vi "libssh2_channel_receive_window_adjust2.vi"(8 "error in (no error)":errorcluster, 9 "force (F)":bool, 10 "adjustment":u32, 11 "channel":T1) -> (0 "error out":errorcluster, 2 "window":u32)   [LabVIEW 2013, in "libssh2.lvlib"]
doc: "Adjust the receive window for a channel by <B>adjustment</B> bytes.\nIf the amount to be adjusted is less than 1024 and <B>force</B> is zero the adjustment amount will be queued for a later packet.\n\nReturns the new size of the receive window."
uses:
  libssh2.lvlib
  Channel Refnum.ctl
  Not A Channel.vi
  <vilib>/Utility/error.llb/Error Cluster From Error Code.vi
  Global Settings.vi
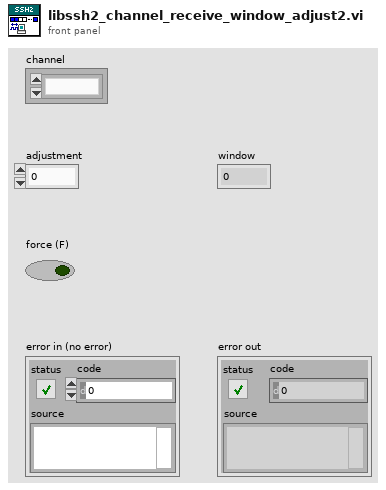
[diagram p1: front panel]
types:
  T1 = typedef "libssh2.lvlib/Channel Refnum.ctl" = refnum<k1>
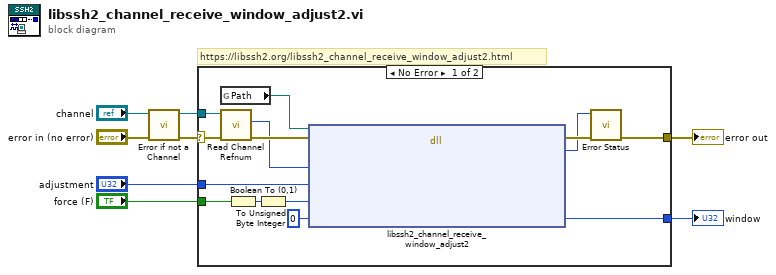
[diagram p0: block diagram]
diagram:
  # "https://libssh2.org/libssh2_channel_receive_window_adjust2.html"
  n1 = call "Error if not a Channel.vi"("error in (no error)"="error in (no error)", "channel"="channel") -> ("error out"=w6:errorcluster, "channel out"=w4:T1)  [unwired: 8 in]
  n2 = case shown="No Error" w6 {
    selector: w6 -> [w22 w23]
    tunnel: [w21 w23] -> w8
    tunnel: w4 -> [w20 _]
    tunnel: "adjustment" -> [w14 _]
    tunnel: "force (F)" -> [w13 _]
    tunnel: [w10 _] -> w1
    frame No Error {
      n3 = global read "Global Settings.vi" "Path"() -> (w16:path)
      n4 = call "Read Channel Refnum.vi"("error in (no error)"=w22, "channel"=w20) -> ("error out"=w18:errorcluster, "LIBSSH2_CHANNEL*"=w17:u64)  [unwired: 8 in]
      n5 = Boolean To (0,1)(Boolean=w13) -> (0, 1=w12:i16)
      n6 = To Unsigned Byte Integer(number=w12) -> (unsigned 8bit integer=w11:u8)
      n7 = dll-call lib="?" fn="libssh2_channel_receive_window_adjust2"(path in=w16, error in=w18, "channel"=w17, "adjustment"=w14, "force"=w11, "window"=u32 0) -> (error out=w19:errorcluster, "return value"=w15:i32, "window"=w10:u32)  [unwired: 4 in, 1 out]
      n8 = call "Error Status.vi"("error in (no error)"=w19, "return value"=w15) -> ("error out"=w21:errorcluster)  [unwired: 8 in, 1 out]
    }
    frame Error {
    }
  }
  "error out" <- w8
  "window" <- w1
